vi "Raw to I16.vi"(8 "error in (no error)":errorcluster, 10 "Raw data":string, 11 "Red Pitaya Digitizer in":refnum<class "Red Pitaya Digitizer.lvclass">) -> (0 "error out":errorcluster, 1 "Current read position":i32, 2 "Data out":i16[][](array[numeric]), 3 "Red Pitaya Digitizer out":refnum<class "Red Pitaya Digitizer.lvclass">, 4 "Finished":bool)   [LabVIEW 2016, in "Red Pitaya Digitizer.lvclass"]
uses:
  Red Pitaya Digitizer.lvclass
  C:/github/NHMFL_Core/Libraries/Instruments/Pulse Driver/Pulse Driver.lvclass
  Instruments/Pulse Driver/Pulse Driver.lvclass/Pulse Driver.ctl
  Instruments/Pulse Driver/Read Current read position.vi
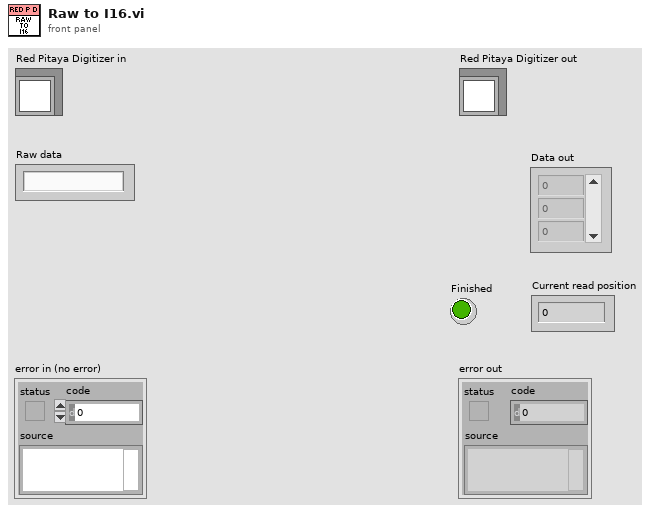
[diagram p1: front panel]
types:
  T1 = enum16{"big-endian, network order", "native, host order", "little-endian"}
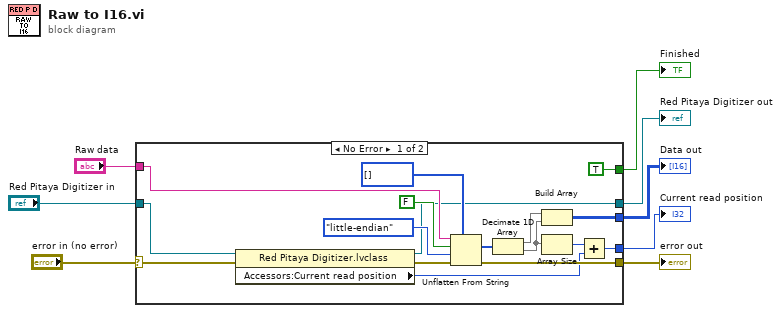
[diagram p0: block diagram]
diagram:
  n1 = case shown="No Error" "error in (no error)" {
    selector: "error in (no error)" -> [w15 w27]
    tunnel: [w18 w27] -> w7
    tunnel: [w9 w26] -> w5
    tunnel: "Red Pitaya Digitizer in" -> [w10 w26]
    tunnel: "Raw data" -> [w17 _]
    tunnel: [w13 _] -> w3
    tunnel: [w12 _] -> w2
    tunnel: [TRUE ("Finished") _] -> w1
    frame No Error {
      n2 = property class="Red Pitaya Digitizer.lvclass"(reference=w10, error in=w15) -> (reference out=w9:refnum<class "Red Pitaya Digitizer.lvclass">, error out=w16:errorcluster, "Accessors:Current read position"=w14:i32)
      n3 = Unflatten From String(type=i16[] [], binary string=w17, data includes array or string size? (T)=FALSE, byte order (0:big-endian, network order)=T1."little-endian", error in (no error)=w16) -> (value=w20:i16[], error out=w18:errorcluster)  [unwired: 1 out]
      n4 = Decimate 1D Array(w20) -> (w19:i16[], w24:i16[])
      n5 = Build Array(w19, w24) -> (w12:i16[][])
      n6 = Array Size(array=w24) -> (size(s)=w25:i32)
      n7 = Add(x=w25, y=w14) -> (x+y=w13:i32)
    }
    frame Error {
    }
  }
  "error out" <- w7
  "Red Pitaya Digitizer out" <- w5
  "Finished" <- w1
  "Current read position" <- w3
  "Data out" <- w2
